vi "CD Add Channel.vi"(8 "error in":errorcluster, 11 "Node Ptr":T1 format="%.0x") -> (0 "error out":errorcluster)   [LabVIEW 2017, in "PXImc System Explorer.lvlib"]
uses:
  PXImc System Explorer.lvlib
  <vilib>/NI Veristand/Custom Device API/Custom Device Item Ref.ctl
  Shared/Channel.ctl
  <vilib>/NI Veristand/Custom Device API/Custom Device Channel Type.ctl
  <vilib>/NI VeriStand/Custom Device API/Custom Device API.lvlib
  Shared/PXImc Shared.lvlib
  <vilib>/NI Veristand/Custom Device Tools/Custom Device Utility Library/Custom Device Utility Library.lvlib
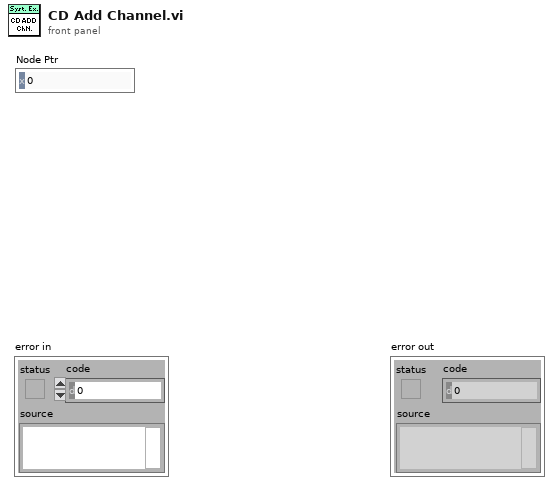
[diagram p1: front panel]
types:
  T1 = typedef "Custom Device API.lvlib/Custom Device Item Ref.ctl" = u64
  T2 = typedef "PXImc Shared.lvlib/Channel.ctl" = cluster{"Name":string, "Units":string, "Default":dbl, "Description":string}
  T3 = typedef "Custom Device API.lvlib/Custom Device Channel Type.ctl" = enum16{"Input", "Output"}
  T4 = typedef "Custom Device API.lvlib/Custom Device Item Info.ctl" = cluster{"Name":string, "Is Channel":bool, "GUID":string, "Is Waveform":bool}
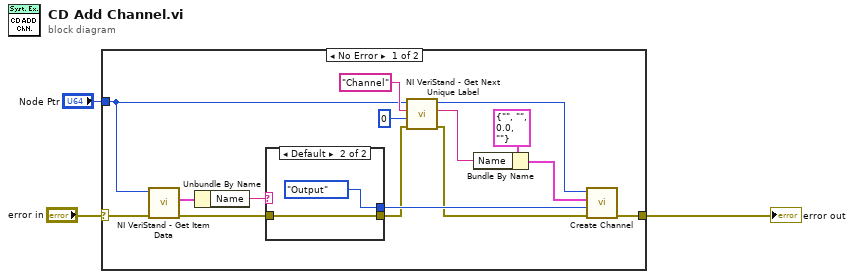
[diagram p0: block diagram]
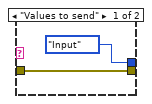
[diagram p2: hidden frame]
diagram:
  n1 = case shown="No Error" "error in" {
    selector: "error in" -> [w16 w23]
    tunnel: [w18 w23] -> w2
    tunnel: "Node Ptr" -> [w6 _]
    frame No Error {
      n2 = call <vilib>:"NI VeriStand - Get Item Data.vi"("error in (no error)"=w16, "Item Ref in"=w6) -> ("error out"=w15:errorcluster, "Item Info"=w17:T4)  [unwired: 6 in, 2 out]
      n3 = Unbundle By Name(w17) -> ("Name"=w14:string)
      n4 = case shown="Default" w14 {
        tunnel: [w20 w22] -> w8
        tunnel: w15 -> [w20 w22]
        tunnel: [Custom_Device_Channel_Type."Input" ("Type") Custom_Device_Channel_Type."Output" ("Type")] -> w13
        frame "Values to send" {
        }
        frame Default {
        }
      }
      n5 = call <vilib>:"NI VeriStand - Get Next Unique Label.vi"("error in (no error)"=w8, "Start Value (1)"=0, "Label"="Channel" ("string"), "Parent Ref in"=w6) -> ("error out"=w7:errorcluster, "Label out"=w9:string, "Parent Ref dup"=w5:T1)  [unwired: 4 in, 1 out]
      n6 = Bundle By Name(cluster=T2 {"Name"="", "Units"="", "Default"=0.0, "Description"=""} ("Channel"), "Name"=w9) -> (w11:T2)
      n7 = call "Create Channel.vi"("error in"=w7, "Type"=w13, "Channel"=w11, "Item Ref in"=w5) -> ("error out"=w18:errorcluster)  [unwired: 6 in, 1 out]
    }
    frame Error {
    }
  }
  "error out" <- w2
